vi "Pigeon Gyro.vi"(2 "Reset to":dbl, 3 "Reset Yaw?":bool) -> (0 "YPR.Yaw Rate":dbl, 1 "YPR.Yaw":dbl)   [LabVIEW 2017, in "Apple script.lvlib"]
uses:
  Apple script.lvlib
  <vilib>/Rock Robotics/WPI/ThirdParty/Phoenix-LabVIEW/Pigeon IMU/CTRE_PigeonIMU_TareType.ctl
  <vilib>/Analysis/baseanly.llb/Mean (DBL).vi
  <vilib>/Rock Robotics/WPI/ThirdParty/Phoenix-LabVIEW/Pigeon IMU/CTRE_PigeonIMU_GetYPR.vi
  <vilib>/Analysis/NI_AALBase.lvlib
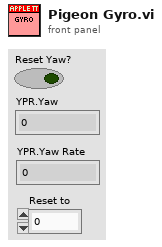
[diagram p1: front panel]
types:
  T1 = typedef "CTRE_PigeonIMU_DeviceRef.ctl" = cluster{"DeviceStatus":errorcluster, "Device Number":u8, "Type":T2, "Device ID":u32, "Handle":u64, "UsageFrame":u32, "Library Path":path}
  T2 = typedef "CTRE_PigeonIMU_ConnectionType.ctl" = u32
  T3 = typedef "CTRE_PigeonIMU_TareType.ctl" = u8
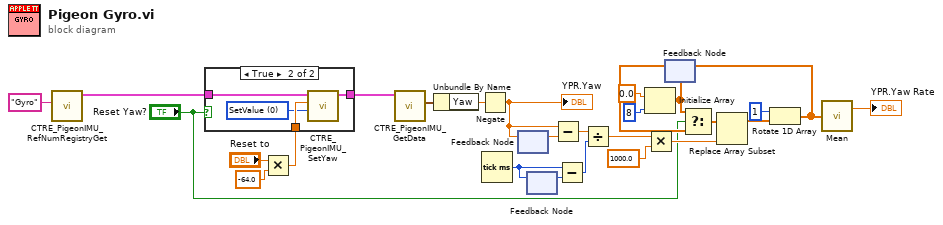
[diagram p0: block diagram]
diagram:
  n1 = call <vilib>:"CTRE_PigeonIMU_RefNumRegistryGet.vi"("refnum name"="Gyro") -> ("PigeonIMUDevRef"=w24:T1)  [unwired: 9 in, 1 out]
  n2 = Multiply(x="Reset to", y=-64.0) -> (x*y=w2:dbl)
  n3 = case shown="True" "Reset Yaw?" {
    tunnel: w24 -> [w28 w32]
    tunnel: w2 -> [_ w31]
    tunnel: [w28 w30] -> w3
    frame False {
    }
    frame True {
      w29 = T3 0 items=["SetValue"=0, "AddOffset"=1, "MatchCompass"=2, "SetOffset"=255] ("TareType (SetValue)")
      n4 = call <vilib>:"CTRE_PigeonIMU_SetYaw.vi"("TareType (SetValue)"=w29, "Value"=w31, "PigeonIMUDevRef"=w32) -> ("PigeonIMUDevRef"=w30:T1)  [unwired: 7 in, 1 out]
    }
  }
  n5 = call-poly <vilib>:"CTRE_PigeonIMU_GetData.vi"("PigeonIMUDevRef"=w3) -> ("Yaw Pitch Roll"=w25:cluster{"Yaw":dbl, "Pitch":dbl, "Roll":dbl})  [unwired: 8 in, 2 out]
  n6 = Unbundle By Name(w25) -> ("Yaw"=w27:dbl)
  n7 = Negate(x=w27) -> (-x=w9:dbl)
  "YPR.Yaw" <- w9
  n8 = Tick Count (ms)() -> (millisecond timer value=w15:u32)
  n9 = feedback #1() -> (w23:dbl)  [unwired: 1 in]
  n10 = feedback-in #1(w9) -> ()
  n11 = feedback #2() -> (w16:u32)  [unwired: 1 in]
  n12 = feedback-in #2(w15) -> ()
  n13 = Subtract(x=w9, y=w23) -> (x-y=w22:dbl)
  n14 = Subtract(x=w15, y=w16) -> (x-y=w14:u32)
  n15 = Divide(x=w22, y=w14) -> (x/y=w10:dbl)
  n16 = Initialize Array(0.0 ("element"), 8 ("dimension size")) -> (w4:dbl[])
  n17 = Multiply(x=w10, y=1000.0 ("x")) -> (x*y=w21:dbl)
  n18 = feedback #3(w4) -> (w18:dbl[])
  n19 = Select(t=w4, s="Reset Yaw?", f=w18) -> (s? t:f=w6:dbl[])
  n20 = Replace Array Subset(array=w6, new element=w21) -> (w20:dbl[])  [unwired: 1 in]
  n21 = Rotate 1D Array(1:w20, 2:1 ("n")) -> (0:w17:dbl[])
  n22 = feedback-in #3(w17) -> ()
  n23 = call-poly <vilib>:"Mean.vi"("X"=w17) -> ("mean"=→"YPR.Yaw Rate":dbl)  [unwired: 1 out]
